vi "test A Future Can Be Cancelled and That State Read By Promise.vi"(8 "error in (no error)":errorcluster, 11 "TestCase in":refnum<class "Cancellation Tests.lvclass">) -> (0 "error out":errorcluster, 3 "TestCase out":refnum<class "Cancellation Tests.lvclass">)   [LabVIEW 2017, in "Cancellation Tests.lvclass"]
uses:
  Cancellation Tests.lvclass
  <vilib>/addons/_JKI Toolkits/VI Tester/TestCase.llb/TestCase.lvclass
  Futures/Futures.lvlib
  Futures/Future/Future.lvclass
  Futures/Promise/Promise.lvclass
  C:/Program Files (x86)/National Instruments/LabVIEW 2017/vi.lib/addons/_JKI Toolkits/VI Tester/TestCase.llb/TestCase.lvclass
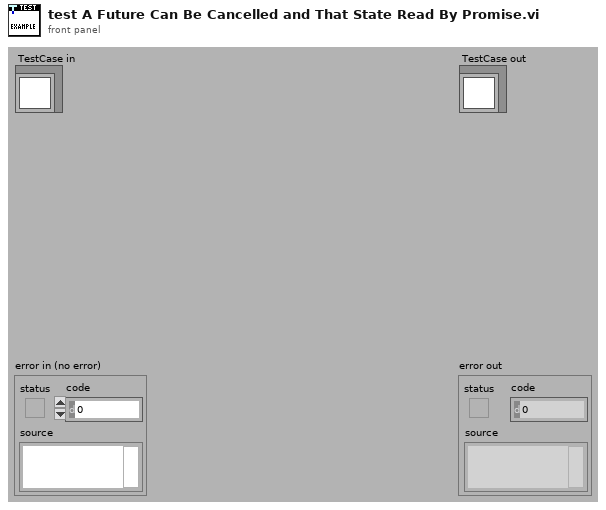
[diagram p1: front panel]
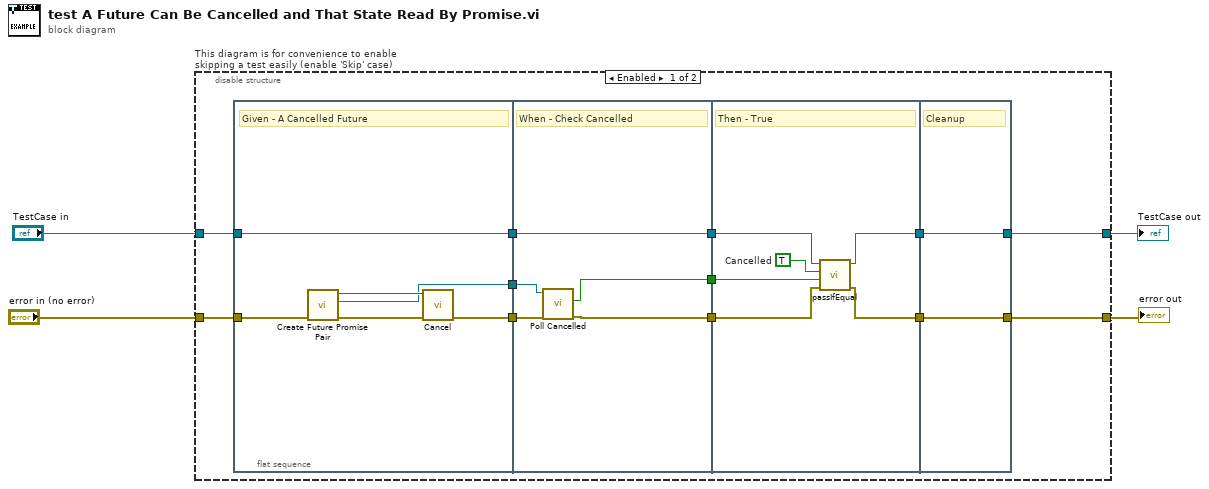
[diagram p0: block diagram]
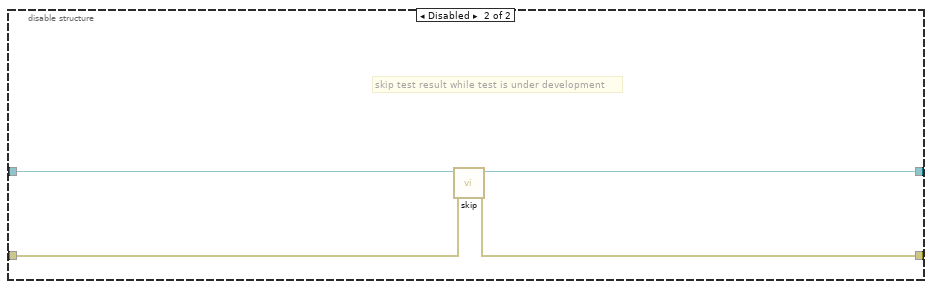
[diagram p2: hidden frame]
diagram:
  n1 = disable-structure "This diagram is for convenience to enable skipping a test easily (enable 'Skip' case)" shown="Enabled" {
    disable-tunnel: "TestCase in" -> [w11 w39]
    disable-tunnel: [w9 w37] -> w1
    disable-tunnel: [w8 w38] -> w3
    disable-tunnel: "error in (no error)" -> [w10 w36]
    frame Enabled {
      n2 = flat-sequence {
        tunnel: w10 -> [w21]
        tunnel: w11 -> [w22]
        tunnel: [w22] -> w16
        tunnel: [w18] -> w7
        tunnel: [w17] -> w6
        tunnel: [w27] -> w15
        tunnel: [w24] -> w14
        tunnel: w16 -> [w27]
        tunnel: w7 -> [w26]
        tunnel: w6 -> [w25]
        tunnel: [w23] -> w5
        tunnel: [w32] -> w13
        tunnel: [w30] -> w12
        tunnel: w15 -> [w33]
        tunnel: w14 -> [w31]
        tunnel: w5 -> [w29]
        tunnel: [w34] -> w8
        tunnel: [w35] -> w9
        tunnel: w13 -> [w35]
        tunnel: w12 -> [w34]
        frame #0 {
          # "Given - A Cancelled Future"
          n3 = call "Create Future Promise Pair.vi"("error in (no error)"=w21) -> ("error out"=w20:errorcluster, "Promise out"=w17:refnum<class "Promise.lvclass">, "Future out"=w19:refnum<class "Future.lvclass">)  [unwired: 8 in]
          n4 = call "Cancel.vi"("error in (no error)"=w20, "Future in"=w19) -> ("error out"=w18:errorcluster)  [unwired: 9 in]
        }
        frame #1 {
          # "When - Check Cancelled"
          n5 = call "Poll Cancelled.vi"("error in (no error)"=w26, "Promise in"=w25) -> ("error out"=w24:errorcluster, "Cancelled"=w23:bool)  [unwired: 7 in, 1 out]
        }
        frame #2 {
          w28 = TRUE  # Cancelled
          # "Then - True"
          n6 = call-dynamic "passIfEqual.vi"("error in (no error)"=w31, "y"=w29, "x"=w28, "TestCase in"=w33) -> ("error out"=w30:errorcluster, "TestCase out"=w32:refnum<class "Cancellation Tests.lvclass">)  [unwired: 6 in]
        }
        frame #3 {
          # "Cleanup"
        }
      }
    }
    frame Disabled {
      # "skip test result while test is under development"
      n7 = call <vilib>:"skip.vi"("error in (no error)"=w36, "TestCase in"=w39) -> ("error out"=w38:errorcluster, "TestCase out"=w37:refnum<class "Cancellation Tests.lvclass">)  [unwired: 8 in]
    }
  }
  "error out" <- w3
  "TestCase out" <- w1
